vi "circ ap.vi"(7 "field":T1, 9 "x_shift":dbl, 10 "y_shift":dbl, 11 "radius":dbl=0.0025) -> (5 "field out":T1)   [LabVIEW 2012, in "LightPipes.lvlib"]
doc: "__declspec(dllexport) void circ_ap(double radius, double y_shift, double x_shift, FIELD* field);"
uses:
  LightPipes.lvlib
  Debug/LightPipes.dll
panel:
  out "error out":errorcluster
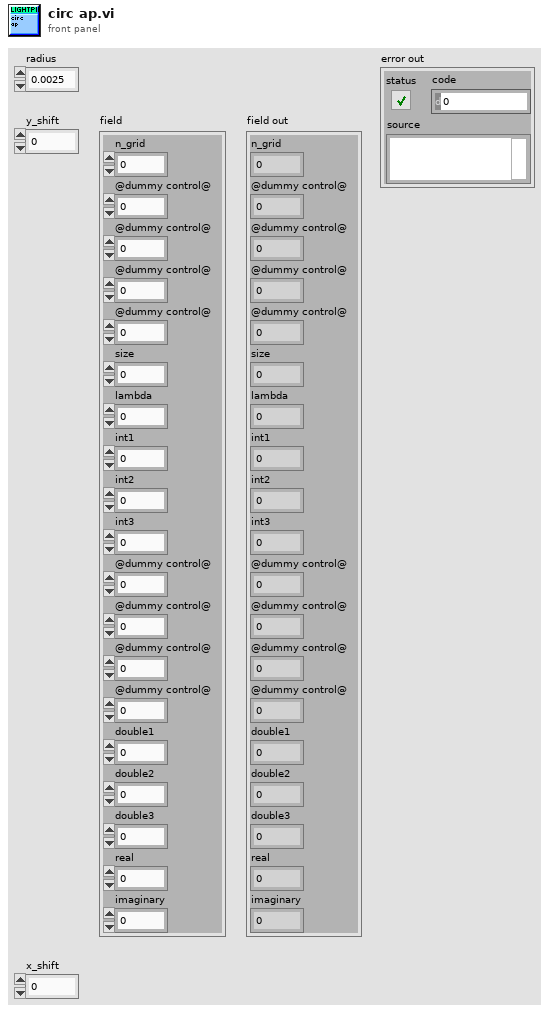
[diagram p1: front panel]
types:
  T1 = cluster{"n_grid":i32, "@dummy control@":i8, "@dummy control@":i8, "@dummy control@":i8, "@dummy control@":i8, "size":dbl, "lambda":dbl, "int1":i32, "int2":i32, "int3":i32, "@dummy control@":i8, "@dummy control@":i8, "@dummy control@":i8, "@dummy control@":i8, "double1":dbl, "double2":dbl, "double3":dbl, "real":u32, "imaginary":u32}
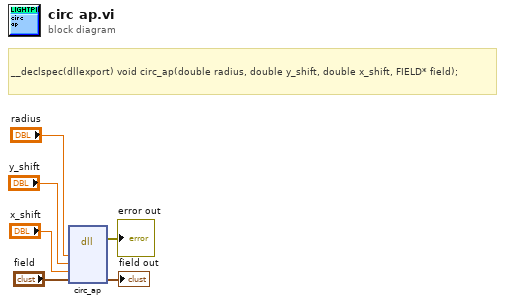
[diagram p0: block diagram]
diagram:
  # "__declspec(dllexport) void circ_ap(double radius, double y_shift, double x_shift, FIELD* field);"
  n1 = dll-call lib="C:/Users/Green Beret/Documents/Visual Studio 2012/Projects/LightPipes/Debug/LightPipes.*" fn="circ_ap"("radius"="radius", "y_shift"="y_shift", "x_shift"="x_shift", "field"="field") -> (error out=→"error out":errorcluster, "field"=→"field out":T1)  [unwired: 7 in, 1 out]
